vi "PatternMatch_FrameShift.vi"(0 "SerRead":string, 3 "StreamingBytesPerFrame":i16=140) -> (4 "foundMatch":bool, 5 "PreStringRemvoed":string, 6 "OutputStr":string, 7 "lengthCorr":i32, 8 "NmissingFromFrame":i32, 9 "NumElRemoved":i32)   [LabVIEW 2020]
panel:
  out "Npartialread":i32
  out "iter":i32
  out "NframesIn":i32
  out "Nframesout":i32
  out "match I":string
  out "firstFrame":string
  out "offset past match kW":i32
  out "after subStr kW":string
  out "match kW":string="\\n "
  out "LengthIn":i32
  out "offset past match":i32
  out "after subStr I":string
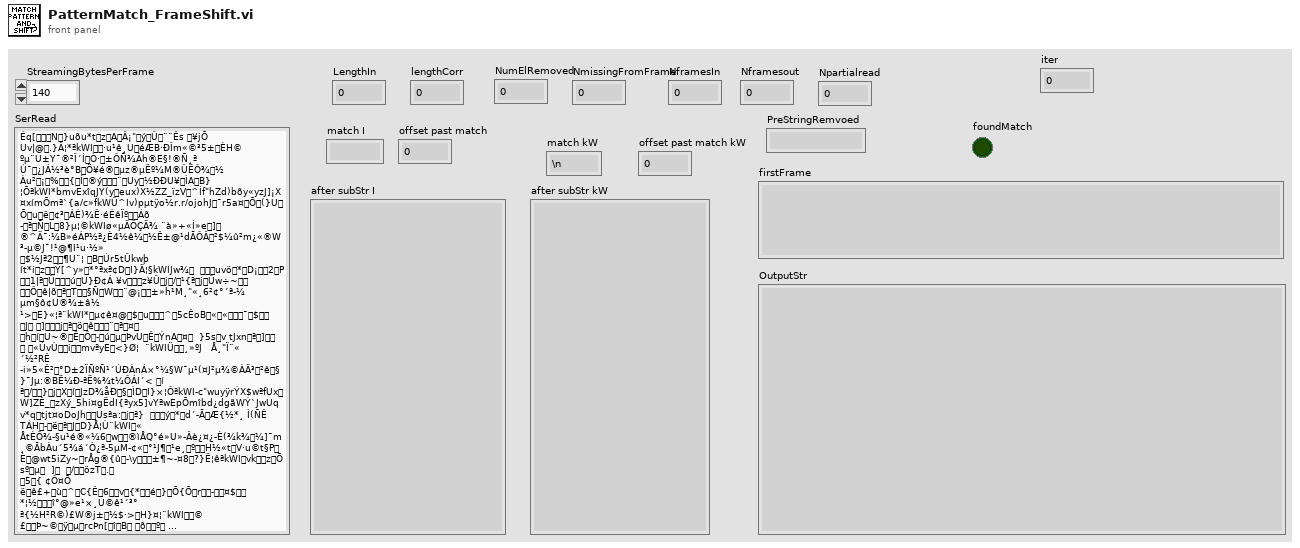
[diagram p1: front panel]
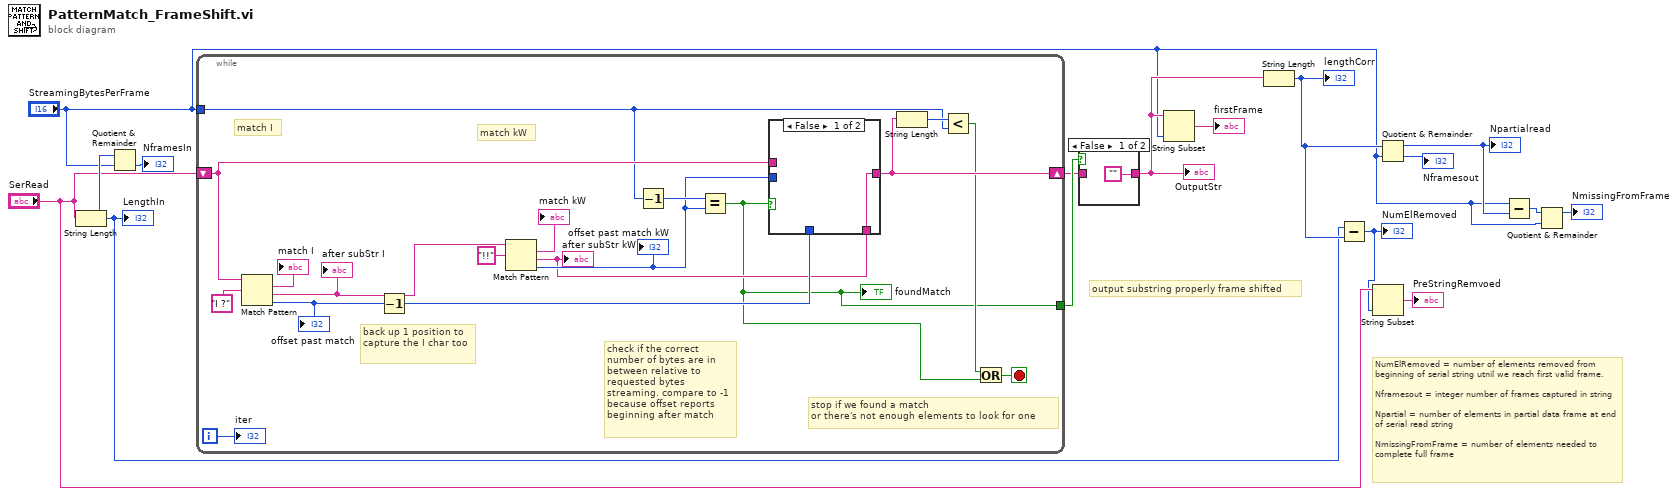
[diagram p0: block diagram]
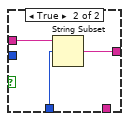
[diagram p3: hidden frame]
diagram:
  # "NumElRemoved = number of elements removed from beginning of serial string utnil we reach first valid frame.\n\nNframesout = integer number of frames captured in string\n\nNpartial = number of elements in partial data frame at end of serial read string\n\nNmissingFromFrame = number of elements needed to complete full frame"
  # "output substring properly frame shifted"
  n1 = String Length(string="SerRead") -> (length=w8:i32)
  "LengthIn" <- w8
  n2 = Quotient & Remainder(x=w8, y="StreamingBytesPerFrame") -> (floor(x/y)=→"NframesIn":i32)  [unwired: 1 out]
  n3 = while {
    tunnel: "StreamingBytesPerFrame" -> [w22]
    shift-right: [w24] -> w11
    shift-left: "SerRead" -> [w29]
    tunnel: [w17] -> w12
    i -> [w25]
    stop <- w20 stop-if-true
    # "stop if we found a match\nor there's not enough elements to look for one"
    # "back up 1 position to capture the I char too"
    # "check if the correct number of bytes are in between relative to requested bytes streaming. compare to -1 because offset reports beginning after match"
    # "match kW"
    # "match I"
    n4 = Match Pattern(string=w29, regular expression="I ?" ("Intan sync byte")) -> (match substring=→"match I":string, after substring=w28:string, offset past match=w31:i32)  [unwired: 1 in, 1 out]
    "after subStr I" <- w28
    "offset past match" <- w31
    n5 = Decrement(x=w31) -> (x-1=w30:i32)
    n6 = Match Pattern(string=w28, regular expression="!!") -> (match substring=→"match kW":string, after substring=w18:string, offset past match=w19:i32)  [unwired: 1 in, 1 out]
    "after subStr kW" <- w18
    "offset past match kW" <- w19
    n7 = Decrement(x=w22) -> (x-1=w27:i16)
    n8 = Equal?(x=w27, y=w19) -> (x = y?=w17:bool)
    "foundMatch" <- w17
    n9 = case shown="False" w17 {
      tunnel: w30 -> [_ w37]
      tunnel: w29 -> [_ w36]
      tunnel: [w34 w35] -> w24
      tunnel: w19 -> [_ _]
      tunnel: w18 -> [w34 _]
      frame False {
      }
      frame True {
        n10 = String Subset(string=w36, offset (0)=w37) -> (substring=w35:string)  [unwired: 1 in]
      }
    }
    n11 = String Length(string=w24) -> (length=w23:i32)
    n12 = Less?(x=w23, y=w22) -> (x < y?=w21:bool)
    n13 = Or(x=w21, y=w17) -> (x .or. y?=w20:bool)
    "iter" <- w25
  }
  n14 = case shown="False" w12 {
    tunnel: w11 -> [_ w39]
    tunnel: ["" w39] -> w10
    frame False {
    }
    frame True {
    }
  }
  "OutputStr" <- w10
  n15 = String Subset(string=w10, length (rest)="StreamingBytesPerFrame") -> (substring=→"firstFrame":string)  [unwired: 1 in]
  n16 = String Length(string=w10) -> (length=w9:i32)
  "lengthCorr" <- w9
  n17 = Subtract(x=w8, y=w9) -> (x-y=w5:i32)
  "NumElRemoved" <- w5
  n18 = String Subset(string="SerRead", length (rest)=w5) -> (substring=→"PreStringRemvoed":string)  [unwired: 1 in]
  n19 = Quotient & Remainder(x=w9, y="StreamingBytesPerFrame") -> (x-y*floor(x/y)=w4:i32, floor(x/y)=→"Nframesout":i32)
  "Npartialread" <- w4
  n20 = Subtract(x="StreamingBytesPerFrame", y=w4) -> (x-y=w2:i32)
  n21 = Quotient & Remainder(x=w2, y="StreamingBytesPerFrame") -> (x-y*floor(x/y)=→"NmissingFromFrame":i32)  [unwired: 1 out]
